vi "Close Instance.vi"(4 "ms timeout (-1)":i32=-1, 8 "error in":errorcluster, 11 "GLue in":refnum<class "class.GLue.lvclass">) -> (0 "error out":errorcluster)   [LabVIEW 2014, in "GLue.lvlib"]
doc: "Closes a previously opened instance of GLue freeing all associated resources.\n\n<B>Parameter(s) </B>\n-----------------\n\n- <B>GLue in:</B> GLue reference to close.\n\n- <B>ms timeout (-1):</B> The time to wait for the GLue reference to become available. A value of '-1' specifies an infinite timeout.\n\n- <B>error in:</B> Describes error conditions that occur before this node runs. This VI runs normally even if an error occurred before this VI runs. \n\n- <B>error out:</B> Contains error information. This output provides standard error out functionality."
uses:
  GLue.lvlib
  Private/Class/class.GLue.lvclass
panel:
  # "Input"
  # "Output"
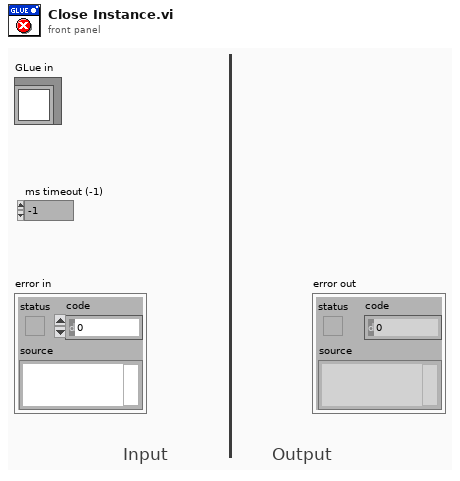
[diagram p1: front panel]
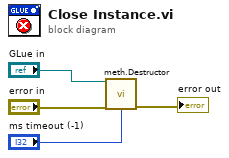
[diagram p0: block diagram]
diagram:
  n1 = call "meth.Destructor.vi"("GLue in"="GLue in", "error in"="error in", "ms timeout (-1)"="ms timeout (-1)") -> ("error out"=→"error out":errorcluster)  [unwired: 12 in]
